vi "Sr830 Read Param.vi"(8 "error in (no error)":errorcluster, 10 "Énum":T1(ring), 11 "Ressource VISA":refnum<visa-resource-name>="SR830A") -> (0 "error out":errorcluster, 2 "Params":string, 3 "Ressource VISA Out":refnum<visa-resource-name>="GPIB0::8::INSTR", 5 "LockInPar":T2={"Phase Shift (°)"=0.0, "Reference Source"=0, "Frequency (Hz)"=0.0, "Reference Trigger"=0, "Harmonic"=0, "Sine Amplitude (V)"=0.0, "Input Configuration"=1, "Input Shield"=0, "Input Coupling"=0, "Input Notch Filters"={"1xLineFilter"=FALSE, "2xLineFilter"=FALSE}, "Sensitivity"=1, "Dynamic Reserve"=0, "Time Constant"=1, "Low Pass Filter"=0, "Sync Filter"=FALSE, "Expand X"={"Offset (%)"=0.0, "Expand"=0}, "Expand Y"={"Offset (%)"=0.0, "Expand"=0}, "Expand R"={"Offset (%)"=0.0, "Expand"=0}} caption="Lock-In Parameters" {"Expand R"."Expand" items=["Off", "x10", "x100"]; "Expand R"."Offset (%)" format="%#.3f"; "Expand Y"."Expand" items=["Off", "x10", "x100"]; "Expand Y"."Offset (%)" format="%#.3f"; "Expand X"."Expand" items=["Off", "x10", "x100"]; "Expand X"."Offset (%)" format="%#.3f"; "Input Coupling" items=["AC", "DC"]; "Input Shield" items=["Float", "Ground"]; "Input Configuration" items=["A", "A-B", "I (1 MOhms)", "I (100 MOhms)", ""]; "Sine Amplitude (V)" format="%#.3f"; "Sensitivity" items=["2 nV/fA", "5 nV/fA", "10 nV/fA", "20 nV/fA", "50 nV/fA", "100 nV/fA", "200 nV/fA", "500 nV/fA", "1 µV/pA", "2 µV/pA", "5 µV/pA", "10 µV/pA", "20 µV/pA", "50 µV/pA", "100µV/pA", "200 µV/pA", "500µV/pA", "1 mV/nA", "2 mV/nA", "5 mV/nA", "10 mV/nA", "20 mV/nA", "50 mV/nA", "100 mV/nA", "200 mV/nA", "500 mV/nA", "1 V/uA"]; "Reference Source" items=["External", "Internal"]; "Phase Shift (°)" format="%#.2f"; "Reference Trigger" items=["Sine Zero Crossing", "TTL Rising Edge", "TTL Falling Edge"]; "Low Pass Filter" items=["6 dB/oct", "12 dB/oct", "18 dB/oct", "24 dB/oct"]; "Time Constant" items=["10 us", "30 us", "100 us", "300 us", "1 ms", "3 ms", "10 ms", "30 ms", "100 ms", "300 ms", "1 s", "3 s", "10 s", "30 s", "100 s", "300 s", "1 ks", "3 ks", "10 ks", "30 ks"]; "Dynamic Reserve" items=["High", "Normal", "Low"]})   [LabVIEW 2019]
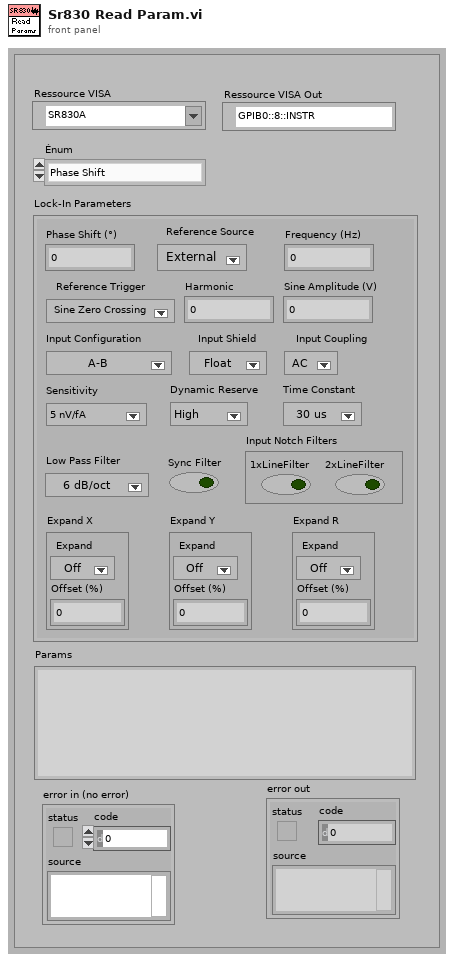
[diagram p1: front panel]
types:
  T1 = enum16{"Phase Shift", "Reference Source", "Reference Frequency", "Reference Trigger", "Detection Harmonic", "Sine Amplitude", "Input Configuration", "Input Shield", "Input Coupling", "Input Line Notch Filter", "Sensitivity", "Dynamic Reserve", "Time Constant", "Low Pass Filter", "Sync Filter", "Expand X", "Expand Y", "Expand R", "All"}
  T2 = cluster{"Phase Shift (°)":dbl, "Reference Source":u16, "Frequency (Hz)":dbl, "Reference Trigger":u16, "Harmonic":i32, "Sine Amplitude (V)":dbl, "Input Configuration":u16, "Input Shield":u16, "Input Coupling":u16, "Input Notch Filters":cluster{"1xLineFilter":bool, "2xLineFilter":bool}, "Sensitivity":u16, "Dynamic Reserve":u16, "Time Constant":u16, "Low Pass Filter":u16, "Sync Filter":bool, "Expand X":cluster{"Offset (%)":dbl, "Expand":u16}, "Expand Y":cluster{"Offset (%)":dbl, "Expand":u16}, "Expand R":cluster{"Offset (%)":dbl, "Expand":u16}}
  T3 = cluster{"Phase Shift (°)":dbl, "Reference Source":u16, "Frequency (Hz)":dbl, "Reference Trigger":u16, "Harmonic":i32, "Sine Amplitude (V)":dbl, "Input Configuration":u16, "Input Shield":u16, "Input Coupling":u16, "Input Notch Filters":cluster{"1xLineFilter":bool, "2xLineFilter":bool}, "Sensitivity":u16, "Dynamic Res.":u16, "Time Constant":u16, "Low Pass Filter":u16, "Sync Filter":bool, "Expand X":cluster{"Offset (%)":dbl, "Expand":u16}, "Expand Y":cluster{"Offset (%)":dbl, "Expand":u16}, "Expand R":cluster{"Offset (%)":dbl, "Expand":u16}}
  T4 = cluster{"Boolean array[0]":bool, "Boolean array[1]":bool}
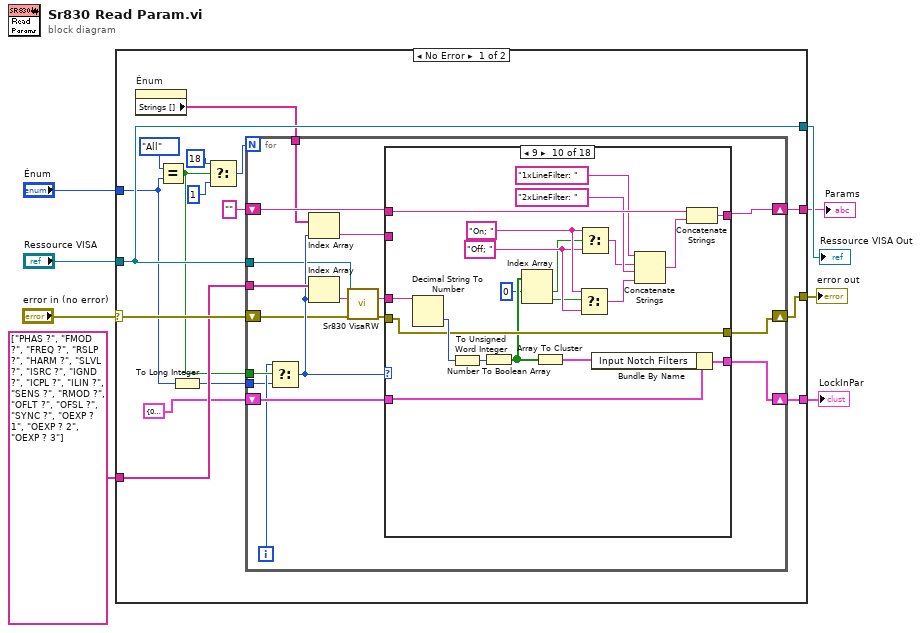
[diagram p0: block diagram]
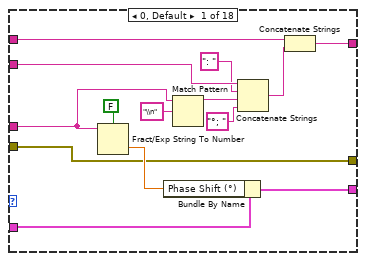
[diagram p2: hidden frame]
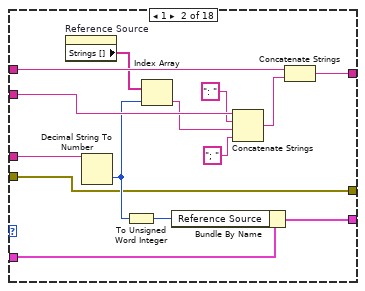
[diagram p3: hidden frame]
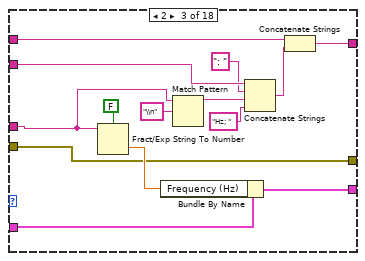
[diagram p4: hidden frame]
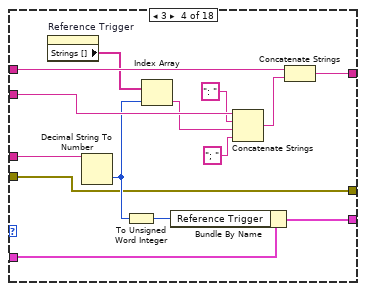
[diagram p5: hidden frame]
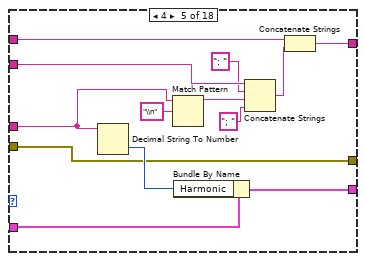
[diagram p6: hidden frame]
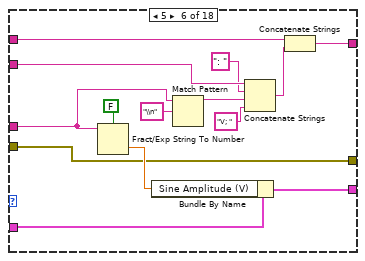
[diagram p7: hidden frame]
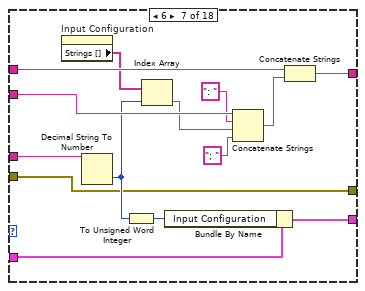
[diagram p8: hidden frame]
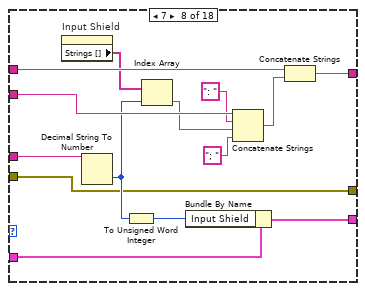
[diagram p9: hidden frame]
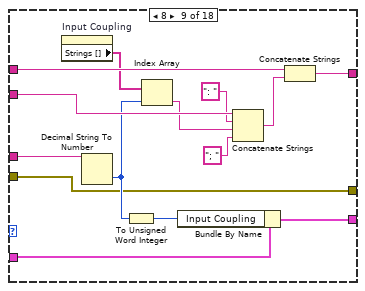
[diagram p10: hidden frame]
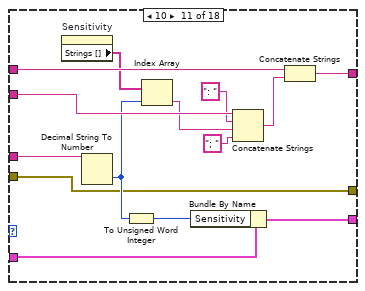
[diagram p11: hidden frame]
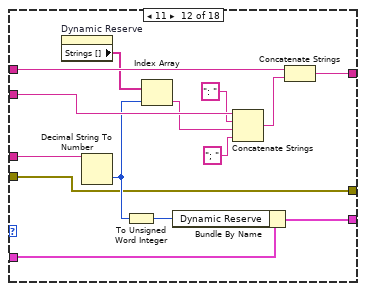
[diagram p12: hidden frame]
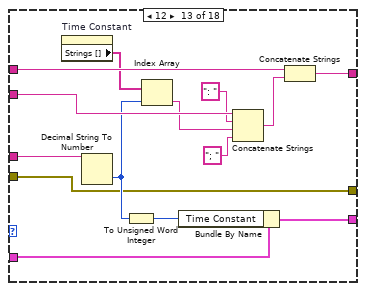
[diagram p13: hidden frame]
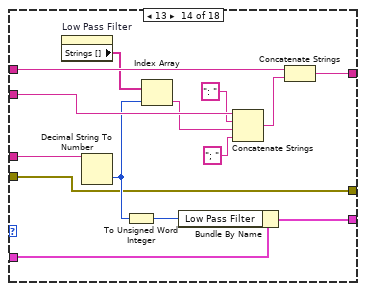
[diagram p14: hidden frame]
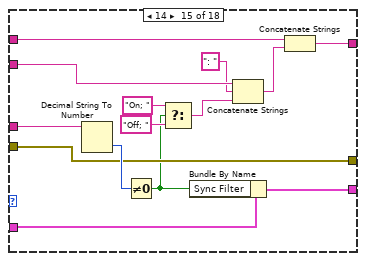
[diagram p15: hidden frame]
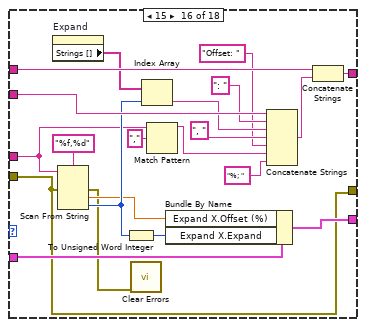
[diagram p16: hidden frame]
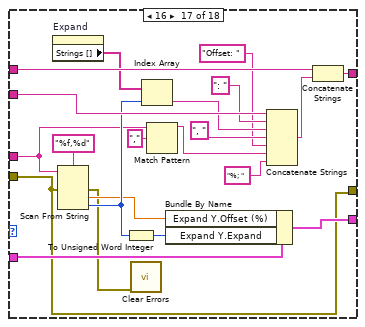
[diagram p17: hidden frame]
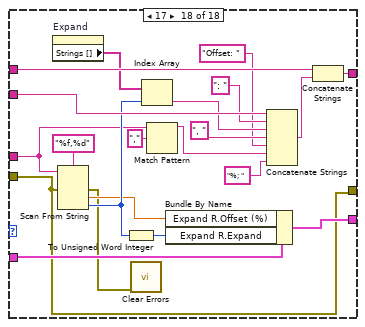
[diagram p18: hidden frame]
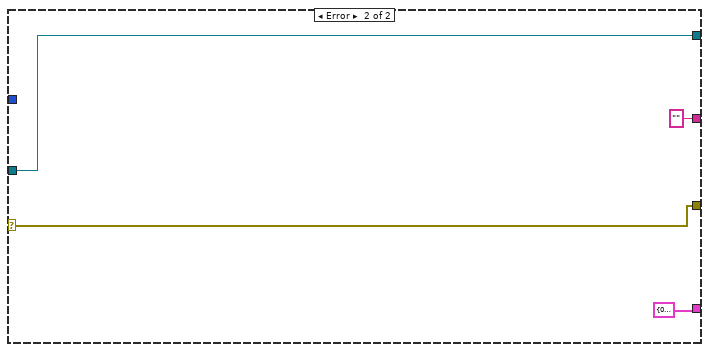
[diagram p19: hidden frame]
diagram:
  n1 = case shown="No Error" "error in (no error)" {
    selector: "error in (no error)" -> [w21 w323]
    tunnel: [w19 w323] -> w7
    tunnel: [w18 w322] -> w6
    tunnel: "Ressource VISA" -> [w18 w322]
    tunnel: "Énum" -> [w13 _]
    tunnel: string[] ["PHAS ?", "FMOD ?", "FREQ ?", "RSLP ?", "HARM ?", "SLVL ?", "ISRC ?", "IGND ?", "ICPL ?", "ILIN ?", "SENS ?", "RMOD ?", "OFLT ?", "OFSL ?", "SYNC ?", "OEXP ? 1", "OEXP ? 2", "OEXP ? 3"] -> [w20 _]
    tunnel: [w16 T3 {"Phase Shift (°)"=0.0, "Reference Source"=0, "Frequency (Hz)"=0.0, "Reference Trigger"=0, "Harmonic"=0, "Sine Amplitude (V)"=0.0, "Input Configuration"=0, "Input Shield"=0, "Input Coupling"=0, "Input Notch Filters"={"1xLineFilter"=FALSE, "2xLineFilter"=FALSE}, "Sensitivity"=0, "Dynamic Res."=0, "Time Constant"=0, "Low Pass Filter"=0, "Sync Filter"=FALSE, "Expand X"={"Offset (%)"=0.0, "Expand"=0}, "Expand Y"={"Offset (%)"=0.0, "Expand"=0}, "Expand R"={"Offset (%)"=0.0, "Expand"=0}} ("LockInPar")] -> w2
    tunnel: [w11 ""] -> w1
    frame No Error {
      n2 = property on="Énum" class="Enum (strict)"() -> ("Strings []"=w15:string[])  [unwired: 2 in, 2 out]
      n3 = Equal?(x=T1."All" ("Énum"), y=w13) -> (x = y?=w14:bool)
      n4 = To Long Integer(number=w13) -> (32bit integer=w12:i32)
      n5 = Select(t=18, s=w14, f=1) -> (s? t:f=w22:i32)
      n6 = for {
        N: w22 -> [_]
        shift-right: [w30] -> w19
        shift-left: w21 -> [w29]
        tunnel: w20 -> [w41]
        tunnel: w18 -> [w27]
        shift-right: [w37] -> w16
        shift-left: T2 {"Phase Shift (°)"=0.0, "Reference Source"=1, "Frequency (Hz)"=0.0, "Reference Trigger"=0, "Harmonic"=0, "Sine Amplitude (V)"=0.0, "Input Configuration"=1, "Input Shield"=0, "Input Coupling"=1, "Input Notch Filters"={"1xLineFilter"=TRUE, "2xLineFilter"=TRUE}, "Sensitivity"=1, "Dynamic Reserve"=0, "Time Constant"=9, "Low Pass Filter"=3, "Sync Filter"=FALSE, "Expand X"={"Offset (%)"=0.0, "Expand"=2}, "Expand Y"={"Offset (%)"=0.0, "Expand"=2}, "Expand R"={"Offset (%)"=0.0, "Expand"=2}} ("LockInPar") -> [w40]
        shift-right: [w39] -> w11
        shift-left: "" -> [w38]
        tunnel: w15 -> [w36]
        tunnel: w14 -> [w34]
        tunnel: w12 -> [w32]
        i -> [w33]
        n7 = Select(t=w33, s=w34, f=w32) -> (s? t:f=w31:i32)
        n8 = Index Array(array=w36, index=w31) -> (element=w35:string)
        n9 = Index Array(array=w41, index=w31) -> (element=w25:string)
        n10 = call <userlib>:"Sr830 VisaRW.vi"("VISA Rsrc"=w27, "ChaineCom"=w25, "error in (no error)"=w29) -> ("ChaineRep"=w26:string, "error out"=w28:errorcluster)  [unwired: 9 in, 2 out]
        n11 = case shown="9" w31 {
          tunnel: w28 -> [w42 w57 w70 w85 w99 w111 w126 w140 w154 w180 w188 w202 w216 w230 w248 w258 w279 w300]
          tunnel: w40 -> [w54 w69 w82 w97 w110 w123 w138 w152 w166 w186 w200 w214 w228 w242 w256 w277 w298 w319]
          tunnel: [w50 w66 w78 w94 w106 w119 w135 w149 w163 w184 w197 w211 w225 w239 w254 w275 w296 w317] -> w39
          tunnel: w38 -> [w49 w65 w77 w93 w105 w118 w134 w148 w162 w183 w196 w210 w224 w238 w253 w274 w295 w316]
          tunnel: [w48 w64 w76 w92 w104 w117 w133 w147 w161 w182 w195 w209 w223 w237 w252 w273 w294 w315] -> w37
          tunnel: w35 -> [w47 w63 w75 w91 w103 w116 w132 w146 w160 _ w194 w208 w222 w236 w251 w272 w293 w314]
          tunnel: [w42 w57 w70 w85 w99 w111 w126 w140 w154 w180 w188 w202 w216 w230 w248 w258 w279 w300] -> w30
          tunnel: w26 -> [w43 w56 w71 w84 w98 w112 w125 w139 w153 w179 w187 w201 w215 w229 w247 w259 w280 w301]
          frame 0, Default {
            n12 = Fract/Exp String To Number(use system decimal point (T)=FALSE ("utiliser le séparateur décimal du système (V)"), string=w43) -> (number=w53:dbl)  [unwired: 2 in, 1 out]
            n13 = Bundle By Name(cluster=w54, "Phase Shift (°)"=w53) -> (w48:T2)
            n14 = Match Pattern(string=w43, regular expression="\\n" ("expression régulière")) -> (before substring=w45:string)  [unwired: 1 in, 3 out]
            n15 = Concatenate Strings(w47, ": " ("chaîne"), w45, "°; " ("chaîne")) -> (w51:string)
            n16 = Concatenate Strings(w49, w51) -> (w50:string)
          }
          frame 1 {
            n17 = property on="Reference Source" class="Ring (strict)"() -> ("Strings []"=w61:string[])  [unwired: 2 in, 2 out]
            n18 = Decimal String To Number(string=w56) -> (number=w60:i32)  [unwired: 2 in, 1 out]
            n19 = To Unsigned Word Integer(number=w60) -> (unsigned 16bit integer=w59:u16)
            n20 = Index Array(array=w61, index=w60) -> (element=w58:string)
            n21 = Bundle By Name(cluster=w69, "Reference Source"=w59) -> (w64:T2)
            n22 = Concatenate Strings(w63, ": " ("chaîne"), w58, "; " ("chaîne")) -> (w67:string)
            n23 = Concatenate Strings(w65, w67) -> (w66:string)
          }
          frame 2 {
            n24 = Fract/Exp String To Number(use system decimal point (T)=FALSE ("utiliser le séparateur décimal du système (V)"), string=w71) -> (number=w81:dbl)  [unwired: 2 in, 1 out]
            n25 = Bundle By Name(cluster=w82, "Frequency (Hz)"=w81) -> (w76:T2)
            n26 = Match Pattern(string=w71, regular expression="\\n" ("expression régulière")) -> (before substring=w73:string)  [unwired: 1 in, 3 out]
            n27 = Concatenate Strings(w75, ": " ("chaîne"), w73, "Hz; " ("chaîne")) -> (w79:string)
            n28 = Concatenate Strings(w77, w79) -> (w78:string)
          }
          frame 3 {
            n29 = property on="Reference Trigger" class="Ring (strict)"() -> ("Strings []"=w89:string[])  [unwired: 2 in, 2 out]
            n30 = Decimal String To Number(string=w84) -> (number=w88:i32)  [unwired: 2 in, 1 out]
            n31 = To Unsigned Word Integer(number=w88) -> (unsigned 16bit integer=w87:u16)
            n32 = Index Array(array=w89, index=w88) -> (element=w86:string)
            n33 = Bundle By Name(cluster=w97, "Reference Trigger"=w87) -> (w92:T2)
            n34 = Concatenate Strings(w91, ": " ("chaîne"), w86, "; " ("chaîne")) -> (w95:string)
            n35 = Concatenate Strings(w93, w95) -> (w94:string)
          }
          frame 4 {
            n36 = Decimal String To Number(string=w98) -> (number=w109:i32)  [unwired: 2 in, 1 out]
            n37 = Match Pattern(string=w98, regular expression="\\n" ("expression régulière")) -> (before substring=w101:string)  [unwired: 1 in, 3 out]
            n38 = Bundle By Name(cluster=w110, "Harmonic"=w109) -> (w104:T2)
            n39 = Concatenate Strings(w103, ": " ("chaîne"), w101, "; " ("chaîne")) -> (w107:string)
            n40 = Concatenate Strings(w105, w107) -> (w106:string)
          }
          frame 5 {
            n41 = Fract/Exp String To Number(use system decimal point (T)=FALSE ("utiliser le séparateur décimal du système (V)"), string=w112) -> (number=w122:dbl)  [unwired: 2 in, 1 out]
            n42 = Bundle By Name(cluster=w123, "Sine Amplitude (V)"=w122) -> (w117:T2)
            n43 = Match Pattern(string=w112, regular expression="\\n" ("expression régulière")) -> (before substring=w114:string)  [unwired: 1 in, 3 out]
            n44 = Concatenate Strings(w116, ": " ("chaîne"), w114, "V; " ("chaîne")) -> (w120:string)
            n45 = Concatenate Strings(w118, w120) -> (w119:string)
          }
          frame 6 {
            n46 = property on="Input Configuration" class="Ring (strict)"() -> ("Strings []"=w130:string[])  [unwired: 2 in, 2 out]
            n47 = Decimal String To Number(string=w125) -> (number=w129:i32)  [unwired: 2 in, 1 out]
            n48 = To Unsigned Word Integer(number=w129) -> (unsigned 16bit integer=w128:u16)
            n49 = Index Array(array=w130, index=w129) -> (element=w127:string)
            n50 = Bundle By Name(cluster=w138, "Input Configuration"=w128) -> (w133:T2)
            n51 = Concatenate Strings(w132, ": " ("chaîne"), w127, "; " ("chaîne")) -> (w136:string)
            n52 = Concatenate Strings(w134, w136) -> (w135:string)
          }
          frame 7 {
            n53 = property on="Input Shield" class="Ring (strict)"() -> ("Strings []"=w144:string[])  [unwired: 2 in, 2 out]
            n54 = Decimal String To Number(string=w139) -> (number=w143:i32)  [unwired: 2 in, 1 out]
            n55 = To Unsigned Word Integer(number=w143) -> (unsigned 16bit integer=w142:u16)
            n56 = Index Array(array=w144, index=w143) -> (element=w141:string)
            n57 = Bundle By Name(cluster=w152, "Input Shield"=w142) -> (w147:T2)
            n58 = Concatenate Strings(w146, ": " ("chaîne"), w141, "; " ("chaîne")) -> (w150:string)
            n59 = Concatenate Strings(w148, w150) -> (w149:string)
          }
          frame 8 {
            n60 = property on="Input Coupling" class="Ring (strict)"() -> ("Strings []"=w158:string[])  [unwired: 2 in, 2 out]
            n61 = Decimal String To Number(string=w153) -> (number=w157:i32)  [unwired: 2 in, 1 out]
            n62 = To Unsigned Word Integer(number=w157) -> (unsigned 16bit integer=w156:u16)
            n63 = Index Array(array=w158, index=w157) -> (element=w155:string)
            n64 = Bundle By Name(cluster=w166, "Input Coupling"=w156) -> (w161:T2)
            n65 = Concatenate Strings(w160, ": " ("chaîne"), w155, "; " ("chaîne")) -> (w164:string)
            n66 = Concatenate Strings(w162, w164) -> (w163:string)
          }
          frame 9 {
            w173 = "Off; " ("chaîne")
            w174 = "On; " ("chaîne")
            n67 = Decimal String To Number(string=w179) -> (number=w181:i32)  [unwired: 2 in, 1 out]
            n68 = To Unsigned Word Integer(number=w181) -> (unsigned 16bit integer=w178:u16)
            n69 = Number To Boolean Array(number=w178) -> (Boolean array=w176:bool[])
            n70 = Index Array(array=w176, index #1=0 ("indice")) -> (element #1=w171:bool, element #2=w172:bool)  [unwired: 1 in]
            n71 = Array To Cluster(array=w176) -> (cluster=w177:T4)
            n72 = Select(t=w174, s=w172, f=w173) -> (s? t:f=w167:string)
            n73 = Select(t=w174, s=w171, f=w173) -> (s? t:f=w168:string)
            n74 = Bundle By Name(cluster=w186, "Input Notch Filters"=w177) -> (w182:T2)
            n75 = Concatenate Strings("1xLineFilter: " ("chaîne"), w168, "2xLineFilter: " ("chaîne"), w167) -> (w185:string)
            n76 = Concatenate Strings(w183, w185) -> (w184:string)
          }
          frame 10 {
            n77 = property on="Sensitivity" class="Ring (strict)"() -> ("Strings []"=w192:string[])  [unwired: 2 in, 2 out]
            n78 = Decimal String To Number(string=w187) -> (number=w191:i32)  [unwired: 2 in, 1 out]
            n79 = To Unsigned Word Integer(number=w191) -> (unsigned 16bit integer=w190:u16)
            n80 = Index Array(array=w192, index=w191) -> (element=w189:string)
            n81 = Bundle By Name(cluster=w200, "Sensitivity"=w190) -> (w195:T2)
            n82 = Concatenate Strings(w194, ": " ("chaîne"), w189, "; " ("chaîne")) -> (w198:string)
            n83 = Concatenate Strings(w196, w198) -> (w197:string)
          }
          frame 11 {
            n84 = property on="Dynamic Reserve" class="Ring (strict)"() -> ("Strings []"=w206:string[])  [unwired: 2 in, 2 out]
            n85 = Decimal String To Number(string=w201) -> (number=w205:i32)  [unwired: 2 in, 1 out]
            n86 = To Unsigned Word Integer(number=w205) -> (unsigned 16bit integer=w204:u16)
            n87 = Index Array(array=w206, index=w205) -> (element=w203:string)
            n88 = Bundle By Name(cluster=w214, "Dynamic Reserve"=w204) -> (w209:T2)
            n89 = Concatenate Strings(w208, ": " ("chaîne"), w203, "; " ("chaîne")) -> (w212:string)
            n90 = Concatenate Strings(w210, w212) -> (w211:string)
          }
          frame 12 {
            n91 = property on="Time Constant" class="Ring (strict)"() -> ("Strings []"=w220:string[])  [unwired: 2 in, 2 out]
            n92 = Decimal String To Number(string=w215) -> (number=w219:i32)  [unwired: 2 in, 1 out]
            n93 = To Unsigned Word Integer(number=w219) -> (unsigned 16bit integer=w218:u16)
            n94 = Index Array(array=w220, index=w219) -> (element=w217:string)
            n95 = Bundle By Name(cluster=w228, "Time Constant"=w218) -> (w223:T2)
            n96 = Concatenate Strings(w222, ": " ("chaîne"), w217, "; " ("chaîne")) -> (w226:string)
            n97 = Concatenate Strings(w224, w226) -> (w225:string)
          }
          frame 13 {
            n98 = property on="Low Pass Filter" class="Ring (strict)"() -> ("Strings []"=w234:string[])  [unwired: 2 in, 2 out]
            n99 = Decimal String To Number(string=w229) -> (number=w233:i32)  [unwired: 2 in, 1 out]
            n100 = To Unsigned Word Integer(number=w233) -> (unsigned 16bit integer=w232:u16)
            n101 = Index Array(array=w234, index=w233) -> (element=w231:string)
            n102 = Bundle By Name(cluster=w242, "Low Pass Filter"=w232) -> (w237:T2)
            n103 = Concatenate Strings(w236, ": " ("chaîne"), w231, "; " ("chaîne")) -> (w240:string)
            n104 = Concatenate Strings(w238, w240) -> (w239:string)
          }
          frame 14 {
            n105 = Decimal String To Number(string=w247) -> (number=w249:i32)  [unwired: 2 in, 1 out]
            n106 = Not Equal To 0?(x=w249) -> (x != 0?=w243:bool)
            n107 = Select(t="On; " ("chaîne"), s=w243, f="Off; " ("chaîne")) -> (s? t:f=w244:string)
            n108 = Bundle By Name(cluster=w256, "Sync Filter"=w243) -> (w252:T2)
            n109 = Concatenate Strings(w251, ": " ("chaîne"), w244) -> (w255:string)
            n110 = Concatenate Strings(w253, w255) -> (w254:string)
          }
          frame 15 {
            n111 = property on="Expand" class="Ring (strict)"() -> ("Strings []"=w270:string[])  [unwired: 2 in, 2 out]
            n112 = Scan From String(format string="%f,%d" ("chaîne de format"), input string=w259, error in=w258) -> (error out=w264:errorcluster, output 1=w265:dbl, output 2=w266:i32)  [unwired: 3 in, 2 out]
            n113 = To Unsigned Word Integer(number=w266) -> (unsigned 16bit integer=w268:u16)
            n114 = call <vilib>:"Clear Errors.vi"("error in (no error)"=w264) -> ()  [unwired: 5 in, 2 out]
            n115 = Index Array(array=w270, index=w266) -> (element=w269:string)
            n116 = Match Pattern(string=w259, regular expression="," ("expression régulière")) -> (before substring=w257:string)  [unwired: 1 in, 3 out]
            n117 = Bundle By Name(cluster=w277, "Expand X.Offset (%)"=w265, "Expand X.Expand"=w268) -> (w273:T2)
            n118 = Concatenate Strings(w272, ": " ("chaîne"), w269, ", " ("chaîne"), "Offset: " ("chaîne"), w257, "%; " ("chaîne")) -> (w276:string)
            n119 = Concatenate Strings(w274, w276) -> (w275:string)
          }
          frame 16 {
            n120 = property on="Expand" class="Ring (strict)"() -> ("Strings []"=w291:string[])  [unwired: 2 in, 2 out]
            n121 = Scan From String(format string="%f,%d" ("chaîne de format"), input string=w280, error in=w279) -> (error out=w285:errorcluster, output 1=w286:dbl, output 2=w287:i32)  [unwired: 3 in, 2 out]
            n122 = To Unsigned Word Integer(number=w287) -> (unsigned 16bit integer=w289:u16)
            n123 = call <vilib>:"Clear Errors.vi"("error in (no error)"=w285) -> ()  [unwired: 5 in, 2 out]
            n124 = Index Array(array=w291, index=w287) -> (element=w290:string)
            n125 = Match Pattern(string=w280, regular expression="," ("expression régulière")) -> (before substring=w278:string)  [unwired: 1 in, 3 out]
            n126 = Bundle By Name(cluster=w298, "Expand Y.Offset (%)"=w286, "Expand Y.Expand"=w289) -> (w294:T2)
            n127 = Concatenate Strings(w293, ": " ("chaîne"), w290, ", " ("chaîne"), "Offset: " ("chaîne"), w278, "%; " ("chaîne")) -> (w297:string)
            n128 = Concatenate Strings(w295, w297) -> (w296:string)
          }
          frame 17 {
            n129 = property on="Expand" class="Ring (strict)"() -> ("Strings []"=w312:string[])  [unwired: 2 in, 2 out]
            n130 = Scan From String(format string="%f,%d" ("chaîne de format"), input string=w301, error in=w300) -> (error out=w306:errorcluster, output 1=w307:dbl, output 2=w308:i32)  [unwired: 3 in, 2 out]
            n131 = To Unsigned Word Integer(number=w308) -> (unsigned 16bit integer=w310:u16)
            n132 = call <vilib>:"Clear Errors.vi"("error in (no error)"=w306) -> ()  [unwired: 5 in, 2 out]
            n133 = Index Array(array=w312, index=w308) -> (element=w311:string)
            n134 = Match Pattern(string=w301, regular expression="," ("expression régulière")) -> (before substring=w299:string)  [unwired: 1 in, 3 out]
            n135 = Bundle By Name(cluster=w319, "Expand R.Offset (%)"=w307, "Expand R.Expand"=w310) -> (w315:T2)
            n136 = Concatenate Strings(w314, ": " ("chaîne"), w311, ", " ("chaîne"), "Offset: " ("chaîne"), w299, "%; " ("chaîne")) -> (w318:string)
            n137 = Concatenate Strings(w316, w318) -> (w317:string)
          }
        }
      }
    }
    frame Error {
    }
  }
  "error out" <- w7
  "Ressource VISA Out" <- w6
  "LockInPar" <- w2
  "Params" <- w1
